vi "acquire_fp_yk_FIFO.vi"(6 "numChannels":i16, 7 "Iters":i32, 8 "error in (no error)":errorcluster, 11 "FPGA Interface":T1) -> (0 "error out":errorcluster, 1 "Elements Remaining":u32, 2 "2D Data Out":dbl[][](array[numeric]), 3 "acquisition done":bool, 5 "u iter":i32)   [LabVIEW 2017, in "fpga_fp_interface.lvlib"]
uses:
  fpga_fp_interface.lvlib
  fpga_interface_types/FPGA_to_HOST_1_fp_FIFO_interface.ctl
  <vilib>/Utility/error.llb/Error Cluster From Error Code.vi
  <vilib>/rvi/errors/niLvFpgaAdjustHostInterfaceError.vi
  <vilib>/rvi/interface/nirviMethod/nirviMethod.xnode
  <vilib>/FPGAPlugInAG/Dynamic/niLvFpga_ReadFifo_Dynamic.vi
  <vilib>/rvi/errors/niLvFpgaMergeErrorWithErrorCode.vi
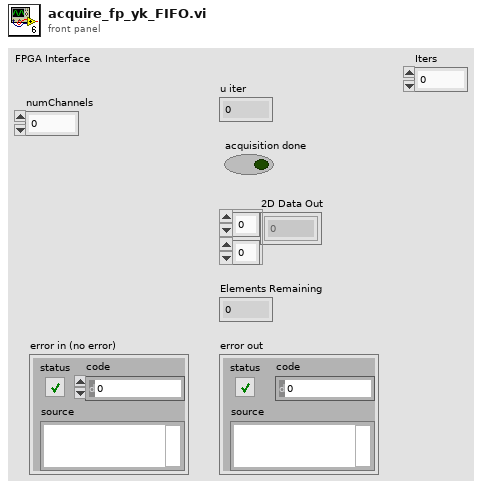
[diagram p1: front panel]
types:
  T1 = typedef "fpga_fp_interface.lvlib/FPGA_to_HOST_1_fp_FIFO_interface.ctl" = refnum<k20>
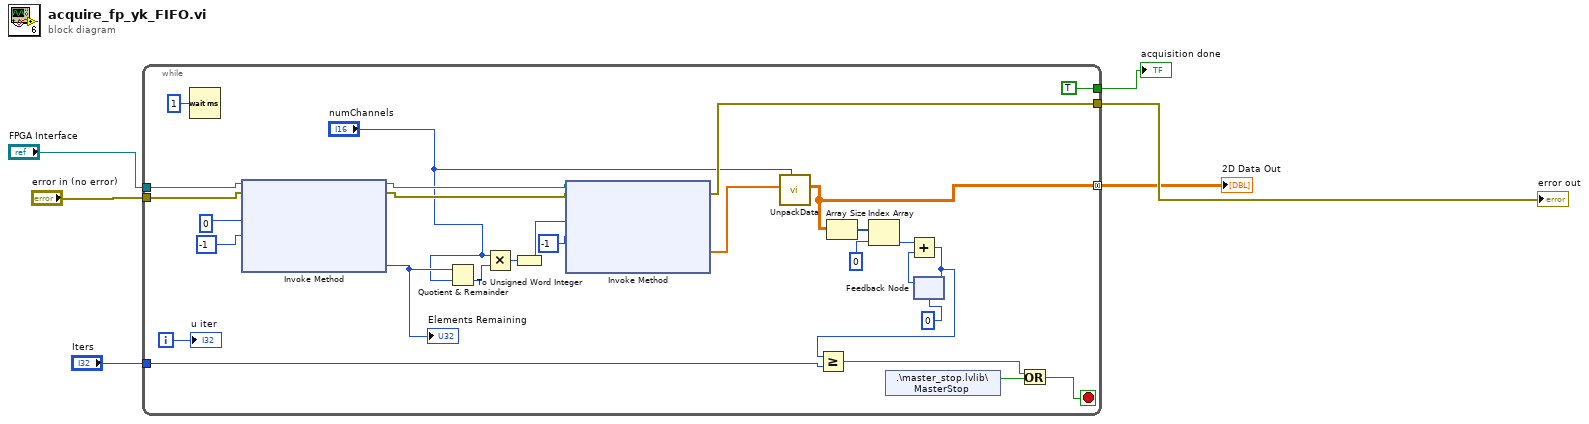
[diagram p0: block diagram]
diagram:
  n1 = while {
    tunnel: [w28] -> w3 mode=concatenating
    tunnel: "FPGA Interface" -> [w22]
    tunnel: "error in (no error)" -> [w21]
    tunnel: [w19] -> w4
    tunnel: [TRUE] -> w6
    tunnel: "Iters" -> [w9]
    i -> [w30]
    stop <- w14 stop-if-true
    n2 = Wait (ms)(milliseconds to wait=u32 1) -> ()  [unwired: 1 out]
    n3 = xnode "Invoke Method"("FPGA VI Reference In"=w22, "error in"=w21, "Number of Elements"=0 ("Timeout (ms)"), "Timeout (ms)"=-1) -> ("FPGA VI Reference Out"=w15:T1, "error out"=w18:errorcluster, "Elements Remaining"=w25:u32)  [unwired: 1 out]
    "Elements Remaining" <- w25
    n4 = Quotient & Remainder(x=w25, y="numChannels") -> (floor(x/y)=w32:u32)  [unwired: 1 out]
    n5 = Multiply(x="numChannels", y=w32) -> (x*y=w33:u32)
    n6 = To Unsigned Word Integer(number=w33) -> (unsigned 16bit integer=w17:u16)
    n7 = xnode "Invoke Method"("FPGA VI Reference In"=w15, "error in"=w18, "Number of Elements"=w17, "Timeout (ms)"=-1) -> ("error out"=w19:errorcluster, "Data"=w20:sgl[])  [unwired: 2 out]
    n8 = call "UnpackData.vi"("NumChannels"="numChannels", "1D Data In"=w20) -> ("2D Data Out"=w28:dbl[][])  [unwired: 8 in, 1 out]
    n9 = Array Size(array=w28) -> (size(s)=w26:i32[])
    n10 = Index Array(array=w26, index=0) -> (element=w29:i32)
    n11 = shared-variable ".\\master_stop.lvlib\\MasterStop"() -> (w12:bool)  [unwired: 1 in, 1 out]
    n12 = feedback #1(0) -> (w31:i32)
    n13 = Add(x=w29, y=w31) -> (x+y=w10:i32)
    n14 = Greater Or Equal?(x=w10, y=w9) -> (x >= y?=w13:bool)
    n15 = feedback-in #1(w10) -> ()
    n16 = Or(x=w13, y=w12) -> (x .or. y?=w14:bool)
    "u iter" <- w30
  }
  "acquisition done" <- w6
  "error out" <- w4
  "2D Data Out" <- w3
